vi "Configure Mode.vi"(8 "Mode? (T: CURR)":bool=TRUE, 9 "error in (no error)":errorcluster, 10 "VISA resource name":refnum<visa-resource-name>) -> (1 "error out":errorcluster, 2 "VISA resource name out":refnum<visa-resource-name>)   [LabVIEW 2019]
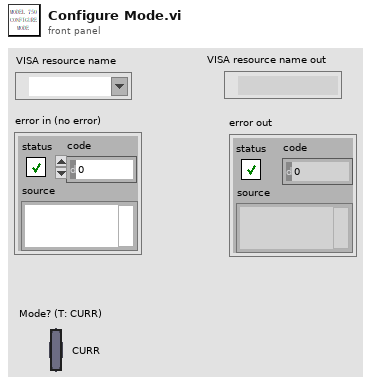
[diagram p1: front panel]
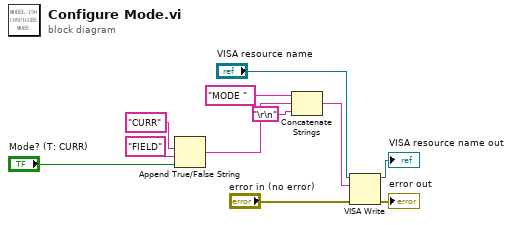
[diagram p0: block diagram]
diagram:
  n1 = Append True/False String(1:"Mode? (T: CURR)", 2:"FIELD", 3:"CURR") -> (0:w2:string)  [unwired: 1 in]
  n2 = Concatenate Strings("MODE " ("字符串"), w2, "\r\n") -> (w8:string)
  n3 = VISA Write(VISA resource name="VISA resource name", write buffer=w8, error in (no error)="error in (no error)") -> (VISA resource name out=→"VISA resource name out":refnum<visa-resource-name>, error out=→"error out":errorcluster)  [unwired: 1 out]
